vi "appendImage.vi"(8 "error in (no error)":errorcluster, 10 "Image Path":path, 11 "MS-Excel in":refnum<class "MS-Excel.lvclass">) -> (0 "error out":errorcluster, 3 "MS-Excel out":refnum<class "MS-Excel.lvclass">)   [LabVIEW 2017, in "LabVIEW NPOI.lvlib" / "MS-Excel.lvclass"]
uses:
  MS-Excel.lvclass
  MS-Excel.lvclass/MS-Excel.ctl
  C:/Users/Neo/Desktop/Dev_Tools_BR/LabVIEW_NPOI/lib/NPOI 2.1.1/NPOI.dll
  lib/NPOI 2.1.1/NPOI.dll
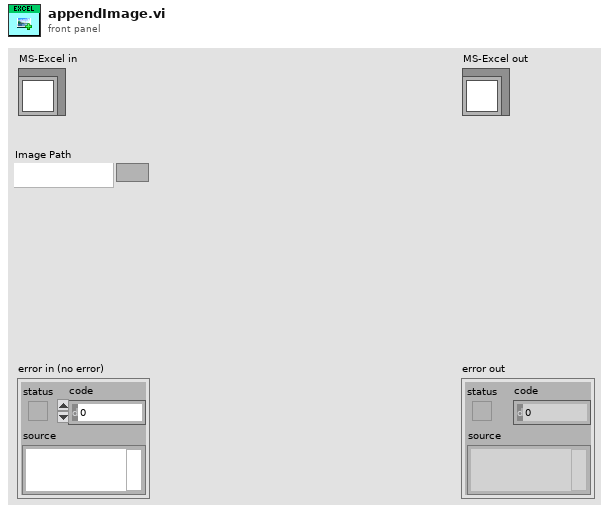
[diagram p1: front panel]
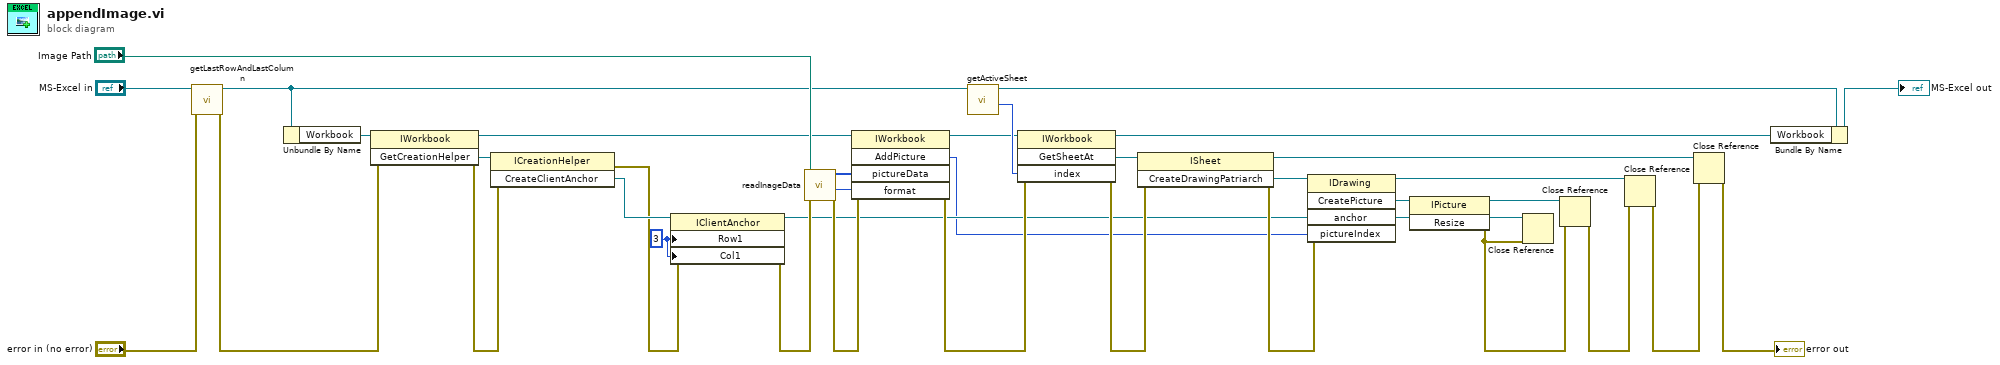
[diagram p0: block diagram]
diagram:
  w4 = 3 ("Row1")
  n1 = call-dynamic "getLastRowAndLastColumn.vi"("error in (no error)"="error in (no error)", "MS-Excel in"="MS-Excel in") -> ("error out"=w21:errorcluster, "MS-Excel out"=w24:refnum<class "MS-Excel.lvclass">)  [unwired: 6 in, 2 out]
  n2 = Unbundle By Name(w24) -> ("Workbook"=w22:refnum<k24>)
  n3 = invoke class="IWorkbook" method="GetCreationHelper"(reference=w22, error in=w21) -> (reference out=w16:refnum<k24>, error out=w20:errorcluster, "GetCreationHelper"=w35:refnum<k24>)  [unwired: 1 in]
  n4 = invoke class="ICreationHelper" method="CreateClientAnchor"(reference=w35, error in=w20) -> (error out=w5:errorcluster, "CreateClientAnchor"=w34:refnum<k24>)  [unwired: 1 in, 1 out]
  n5 = property class="IClientAnchor"(reference=w34, error in=w5, "Row1"=w4, "Col1"=w4) -> (reference out=w15:refnum<k24>, error out=w19:errorcluster)
  n6 = call "readInageData.vi"("error in (no error)"=w19, "file (use dialog)"="Image Path") -> ("error out"=w18:errorcluster, "format"=w26:i32, "Bytes"=w32:u8[])  [unwired: 7 in]
  n7 = invoke class="IWorkbook" method="AddPicture"(reference=w16, error in=w18, "pictureData"=w32, "format"=w26) -> (reference out=w3:refnum<k24>, error out=w17:errorcluster, "AddPicture"=w2:i32)  [unwired: 1 in, 2 out]
  n8 = call-dynamic "getActiveSheet.vi"("MS-Excel in"=w24) -> ("SheetIndex"=w6:i32, "MS-Excel out"=w7:refnum<class "MS-Excel.lvclass">)  [unwired: 7 in, 2 out]
  n9 = invoke class="IWorkbook" method="GetSheetAt"(reference=w3, error in=w17, "index"=w6) -> (reference out=w27:refnum<k24>, error out=w31:errorcluster, "GetSheetAt"=w36:refnum<k24>)  [unwired: 1 in, 1 out]
  n10 = invoke class="ISheet" method="CreateDrawingPatriarch"(reference=w36, error in=w31) -> (reference out=w11:refnum<k24>, error out=w29:errorcluster, "CreateDrawingPatriarch"=w33:refnum<k24>)  [unwired: 1 in]
  n11 = invoke class="IDrawing" method="CreatePicture"(reference=w33, error in=w29, "anchor"=w15, "pictureIndex"=w2) -> (reference out=w12:refnum<k24>, "CreatePicture"=w14:refnum<k24>)  [unwired: 1 in, 3 out]
  n12 = invoke class="IPicture" method="Resize"(reference=w14) -> (reference out=w13:refnum<k24>, error out=w1:errorcluster)  [unwired: 2 in, 1 out]
  n13 = Close Reference(reference=w15, error in (no error)=w1) -> ()  [unwired: 1 out]
  n14 = Close Reference(reference=w13, error in (no error)=w1) -> (error out=w9:errorcluster)
  n15 = Close Reference(reference=w12, error in (no error)=w9) -> (error out=w10:errorcluster)
  n16 = Close Reference(reference=w11, error in (no error)=w10) -> (error out=→"error out":errorcluster)
  n17 = Bundle By Name(cluster=w7, "Workbook"=w27) -> (→"MS-Excel out":refnum<class "MS-Excel.lvclass">)
